vi "Auto limits.vi"(4 "lower band factor":dbl=0.2, 5 "upper band factor":dbl=0.2, 6 "Minimum half range is absolute":bool=TRUE, 7 "Method":string(combo)="interquartile", 8 "Minimum half range":dbl=0.2, 9 "# of interquartile range or stdev":dbl=1.0, 10 "Length":i32=1000, 11 "Input array":dbl[](array[numeric])) -> (0 "Low limit":dbl, 2 "Moving average":dbl, 3 "High limit":dbl)   [LabVIEW 2018]
uses:
  <vilib>/Analysis/baseanly.llb/Mean (DBL).vi
  <vilib>/Analysis/NI_AALBase.lvlib
  <vilib>/gmath/NI_Gmath.lvlib
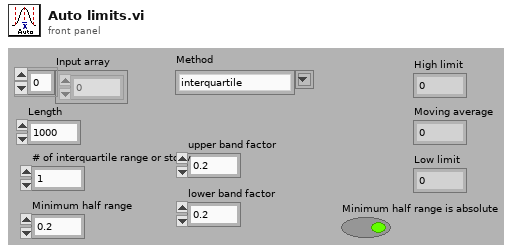
[diagram p1: front panel]
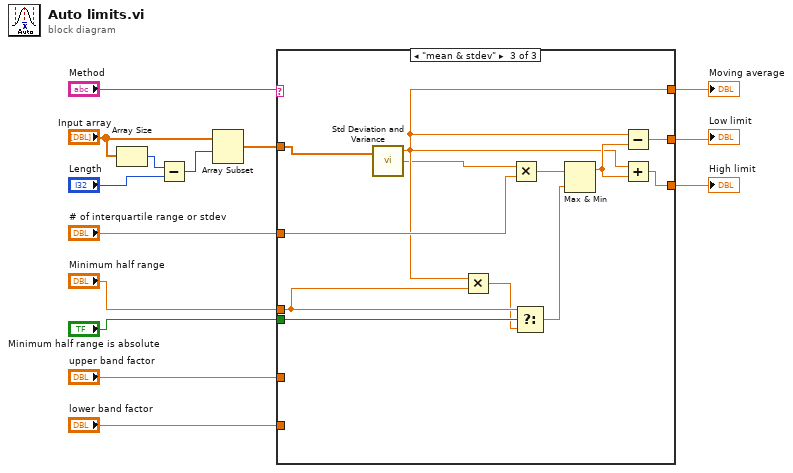
[diagram p0: block diagram]
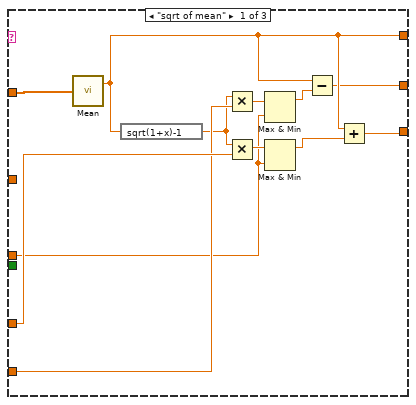
[diagram p2: hidden frame]
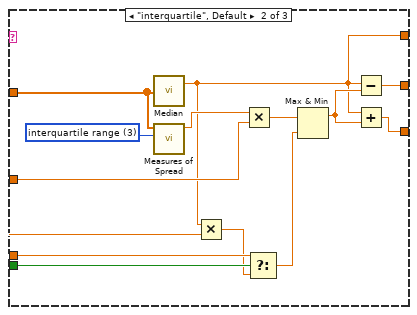
[diagram p3: hidden frame]
diagram:
  n1 = Array Size(array="Input array") -> (size(s)=w13:i32)
  n2 = Subtract(x=w13, y="Length") -> (x-y=w12:i32)
  n3 = Array Subset(array="Input array", index=w12) -> (w7:dbl[])  [unwired: 1 in]
  n4 = case shown="\"mean & stdev\"" "Method" {
    tunnel: "# of interquartile range or stdev" -> [_ w39 w51]
    tunnel: [w20 w36 w48] -> w9
    tunnel: [w24 w35 w47] -> w8
    tunnel: w7 -> [w26 w33 w46]
    tunnel: "Minimum half range is absolute" -> [_ w31 w45]
    tunnel: "Minimum half range" -> [w15 w29 w43]
    tunnel: [w21 w27 w41] -> w4
    tunnel: "upper band factor" -> [w25 _ _]
    tunnel: "lower band factor" -> [w23 _ _]
    frame "sqrt of mean" {
      n5 = call-poly <vilib>:"Mean.vi"("X"=w26) -> ("mean"=w21:dbl)  [unwired: 1 out]
      n6 = expression code="sqrt(1+x)-1"(w21) -> (w22:dbl)
      n7 = Multiply(x=w22, y=w23) -> (x*y=w19:dbl)
      n8 = Multiply(x=w22, y=w25) -> (x*y=w17:dbl)
      n9 = Max & Min(x=w19, y=w15) -> (max(x,y)=w18:dbl)  [unwired: 1 out]
      n10 = Max & Min(x=w17, y=w15) -> (max(x,y)=w16:dbl)  [unwired: 1 out]
      n11 = Subtract(x=w21, y=w18) -> (x-y=w20:dbl)
      n12 = Add(x=w21, y=w16) -> (x+y=w24:dbl)
    }
    frame "interquartile", Default {
      w34 = 3 items=["standard deviation", "range", "mean absolute deviation", "interquartile range"] ("type")
      n13 = call <vilib>:"Median.vi"("X"=w33) -> ("median"=w27:dbl)  [unwired: 1 out]
      n14 = call <vilib>:"Measures of Spread.vi"("type"=w34, "x array"=w33) -> ("spread value"=w32:dbl)  [unwired: 8 in, 1 out]
      n15 = Multiply(x=w27, y=w29) -> (x*y=w28:dbl)
      n16 = Multiply(x=w32, y=w39) -> (x*y=w38:dbl)
      n17 = Select(t=w29, s=w31, f=w28) -> (s? t:f=w30:dbl)
      n18 = Max & Min(x=w38, y=w30) -> (max(x,y)=w37:dbl)  [unwired: 1 out]
      n19 = Subtract(x=w27, y=w37) -> (x-y=w36:dbl)
      n20 = Add(x=w27, y=w37) -> (x+y=w35:dbl)
    }
    frame "mean & stdev" {
      n21 = call <vilib>:"Std Deviation and Variance.vi"("X"=w46) -> ("mean"=w41:dbl, "standard deviation"=w40:dbl)  [unwired: 1 in, 1 out]
      n22 = Multiply(x=w41, y=w43) -> (x*y=w42:dbl)
      n23 = Multiply(x=w40, y=w51) -> (x*y=w50:dbl)
      n24 = Select(t=w43, s=w45, f=w42) -> (s? t:f=w44:dbl)
      n25 = Max & Min(x=w50, y=w44) -> (max(x,y)=w49:dbl)  [unwired: 1 out]
      n26 = Subtract(x=w41, y=w49) -> (x-y=w48:dbl)
      n27 = Add(x=w41, y=w49) -> (x+y=w47:dbl)
    }
  }
  "Low limit" <- w9
  "High limit" <- w8
  "Moving average" <- w4
